vi "spEVENTLOG Send Message.vi"(8 "error in (no error)":errorcluster, 11 "Message (\"\")":string) -> (0 "error out":errorcluster)   [LabVIEW 2011]
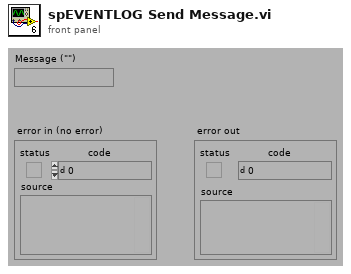
[diagram p1: front panel]
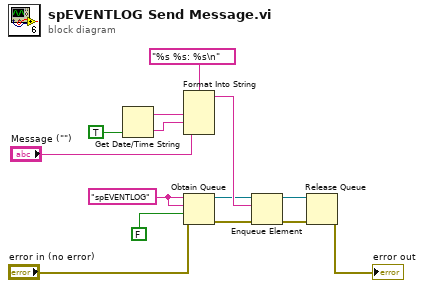
[diagram p0: block diagram]
diagram:
  w7 = "spEVENTLOG"
  n1 = Get Date/Time String(want seconds? (F)=TRUE) -> (date string=w12:string, time string=w13:string)  [unwired: 2 out]
  n2 = Format Into String(format string="%s %s: %s\n", w12, w13, "Message (\"\")") -> (resulting string=w14:string)  [unwired: 2 in, 1 out]
  n3 = Obtain Queue(name (unnamed)=w7, element data type=w7, create if not found? (T)=FALSE, error in (no error)="error in (no error)") -> (queue out=w5:refnum<queue>, error out=w4:errorcluster)  [unwired: 1 in, 1 out]
  n4 = Enqueue Element(queue=w5, element=w14, error in (no error)=w4) -> (queue out=w3:refnum<queue>, error out=w2:errorcluster)  [unwired: 2 out]
  n5 = Release Queue(queue=w3, error in (no error)=w2) -> (error out=→"error out":errorcluster)  [unwired: 1 in, 2 out]
